vi "LVClass_ModalCoef Read ModalCoef.vi"(8 "error in (no error)":errorcluster, 11 "ModalCoef in":refnum<class "ModalCoef.lvclass">) -> (0 "error out":errorcluster, 2 "ModalCoef":T1, 3 "ModalCoef out":refnum<class "ModalCoef.lvclass">)   [LabVIEW 2020, in "ModalCoef.lvclass"]
uses:
  ModalCoef.lvclass
  ClassID.ctl
  ModalCoef.lvclass/ModalCoef.ctl
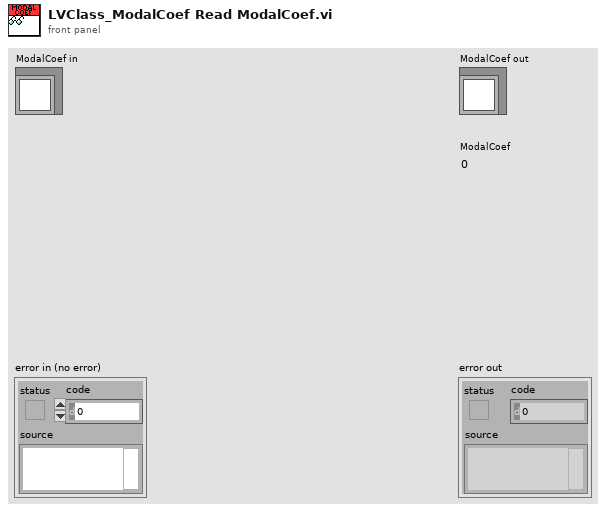
[diagram p1: front panel]
types:
  T1 = typedef "ClassID.ctl" = i64
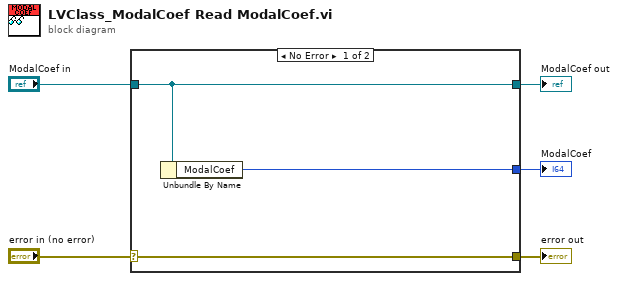
[diagram p0: block diagram]
diagram:
  n1 = case shown="No Error" "error in (no error)" {
    selector: "error in (no error)" -> [w8 w9]
    tunnel: [w8 w9] -> w4
    tunnel: [w7 w10] -> w2
    tunnel: "ModalCoef in" -> [w7 w10]
    tunnel: [w6 _] -> w1
    frame No Error {
      n2 = Unbundle By Name(w7) -> ("ModalCoef"=w6:T1)
    }
    frame Error {
    }
  }
  "error out" <- w4
  "ModalCoef out" <- w2
  "ModalCoef" <- w1
